vi "Get Strings from Ref.vi"(8 "error in (no error)":errorcluster, 9 "Label Prefix":string, 10 "GObj Refnum in":refnum<vi>, 11 "WaveformGraph in":refnum<class "IntensityGraph.lvclass">) -> (0 "error out":errorcluster, 1 "Valid?":bool, 2 "GObj Refnum out":refnum<vi>, 3 "WaveformGraph out":refnum<class "IntensityGraph.lvclass">, 4 "GObj Name":string)   [LabVIEW 2013, in "SET Project Data.lvlib" / "IntensityGraph.lvclass"]
uses:
  IntensityGraph.lvclass
  GraphChart/GraphChart.lvclass
  GObject/GObject.lvclass/GObject.ctl
  GObject/Write UID.vi
  SET Project Data.lvlib
  GObject/GObject.lvclass
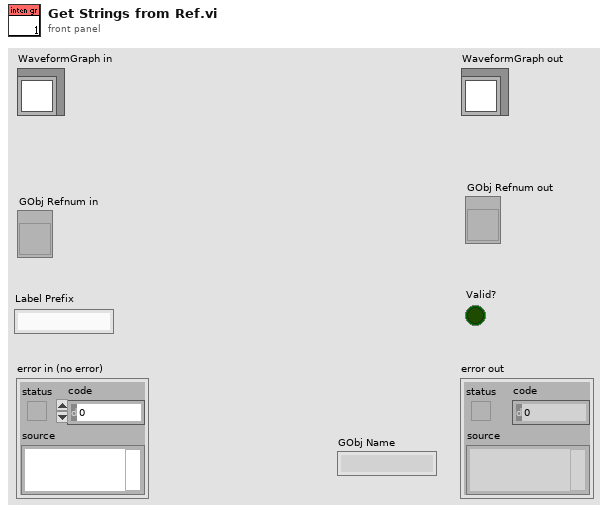
[diagram p1: front panel]
types:
  T1 = typedef "LVCursorListTypeDef.ctl" = cluster{"Name":string, "Color":u32, "Style":u8, "Point Style":u8, "Name Visible":bool, "Allow Drag":bool, "Cursor Mode":u32, "Plot":i32, "Index":i32, "Position":cluster{"X":dbl, "Y":dbl}, "X Scale":u32, "Y Scale":u32, "Watch Plots":i32[], "Watch All Plots":bool, "Plot Area":i32, "Label Offset":cluster{"X":dbl, "Y":dbl}}[]
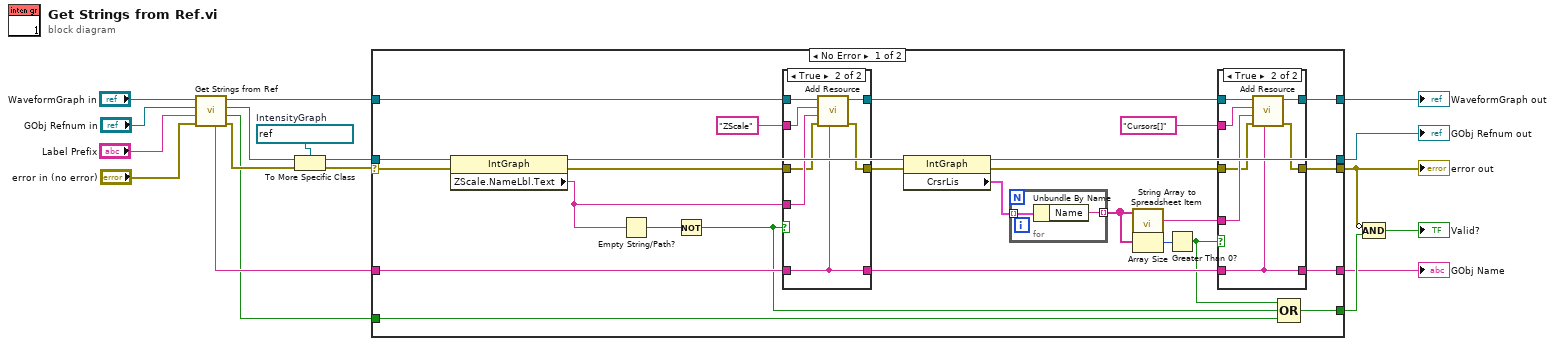
[diagram p0: block diagram]
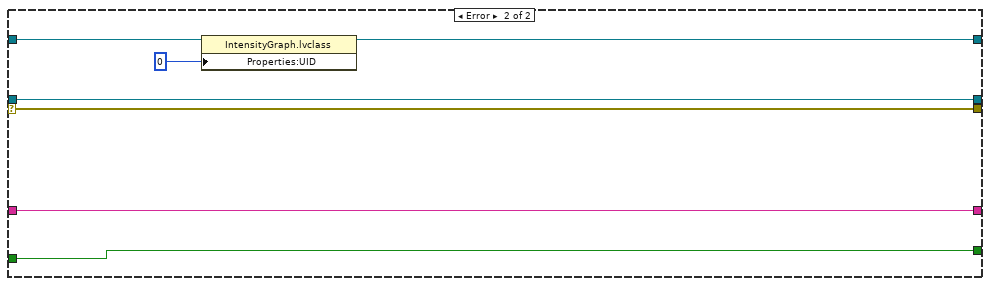
[diagram p4: hidden frame]
diagram:
  w13 = refnum<vi> refnum  # IntensityGraph
  n1 = call-parent "Get Strings from Ref.vi"("error in (no error)"="error in (no error)", "Label Prefix"="Label Prefix", "GObj Refnum in"="GObj Refnum in", "GraphChart in"="WaveformGraph in") -> ("error out"=w9:errorcluster, "Valid?"=w7:bool, "GObj Refnum out"=w10:refnum<vi>, "GraphChart out"=w11:refnum<class "IntensityGraph.lvclass">, "GObj Name"=w8:string)  [unwired: 3 in]
  n2 = To More Specific Class(target class=w13, reference=w10, error in=w9) -> (specific class reference=w6:refnum<vi>, error out=w12:errorcluster)
  n3 = case shown="No Error" w12 {
    selector: w12 -> [w24 w72]
    tunnel: w6 -> [w25 w73]
    tunnel: w11 -> [w43 w71]
    tunnel: [w33 w69] -> w5
    tunnel: [w26 w72] -> w2
    tunnel: [w35 w73] -> w4
    tunnel: w8 -> [w41 w68]
    tunnel: w7 -> [w40 w67]
    tunnel: [w29 w68] -> w1
    tunnel: [w39 w67] -> w14
    frame No Error {
      n4 = property class="IntGraph"(reference=w25, error in=w24) -> (reference out=w22:refnum<vi>, error out=w23:errorcluster, "ZScale.NameLbl.Text"=w21:string)
      n5 = Empty String/Path?(string/path=w21) -> (empty?=w20:bool)
      n6 = Not(x=w20) -> (.not. x?=w19:bool)
      n7 = case shown="True" w19 {
        tunnel: w43 -> [w59 w66]
        tunnel: [w59 w65] -> w34
        tunnel: w41 -> [w58 w62]
        tunnel: w21 -> [_ w64]
        tunnel: "ZScale" -> [_ w63]
        tunnel: [w58 w62] -> w30
        tunnel: w23 -> [w57 w61]
        tunnel: [w57 w60] -> w38
        frame False {
        }
        frame True {
          n8 = call "Add Resource.vi"("TagPrefix"=w62, "error in (no error)"=w61, "ItemText"=w64, "ItemName"=w63, "GObject in"=w66) -> ("error out"=w60:errorcluster, "GObject out"=w65:refnum<class "IntensityGraph.lvclass">)  [unwired: 5 in]
        }
      }
      n9 = property class="IntGraph"(reference=w22, error in=w38) -> (reference out=w35:refnum<vi>, error out=w36:errorcluster, "CrsrLis"=w37:T1)
      n10 = for {
        tunnel: w37 -> [w56] mode=indexing
        tunnel: [w55] -> w28 mode=indexing
        n11 = Unbundle By Name(w56) -> ("Name"=w55:string)
      }
      n12 = call "String Array to Spreadsheet Item.vi"("Strings [] (ASCII)"=w28) -> ("Spreadsheet Item (ASCII)"=w31:string)  [unwired: 10 in]
      n13 = Array Size(array=w28) -> (size(s)=w44:i32)
      n14 = Greater Than 0?(x=w44) -> (x > 0?=w27:bool)
      n15 = case shown="True" w27 {
        tunnel: w34 -> [w47 w54]
        tunnel: [w47 w53] -> w33
        tunnel: w30 -> [w46 w50]
        tunnel: w31 -> [_ w52]
        tunnel: "Cursors[]" -> [_ w51]
        tunnel: [w46 w50] -> w29
        tunnel: w36 -> [w45 w49]
        tunnel: [w45 w48] -> w26
        frame False {
        }
        frame True {
          n16 = call "Add Resource.vi"("TagPrefix"=w50, "error in (no error)"=w49, "ItemText"=w52, "ItemName"=w51, "GObject in"=w54) -> ("error out"=w48:errorcluster, "GObject out"=w53:refnum<class "IntensityGraph.lvclass">)  [unwired: 5 in]
        }
      }
      n17 = Compound Arithmetic op=OR(w27, w19, w40) -> (w39:bool)
    }
    frame Error {
      n18 = property class="IntensityGraph.lvclass"(reference=w71, "Properties:UID"=0 ("UID")) -> (reference out=w69:refnum<class "IntensityGraph.lvclass">)  [unwired: 1 in, 1 out]
    }
  }
  "error out" <- w2
  "WaveformGraph out" <- w5
  "GObj Refnum out" <- w4
  "GObj Name" <- w1
  n19 = Compound Arithmetic op=AND(invert w2, w14) -> (→"Valid?":bool)
